vi "reLU.vi"(9 "Derivative?":bool, 11 "Input":dbl[](array[numeric])) -> (10 "Output":dbl[](array[numeric]))   [LabVIEW 2016]
panel:
  # "reLU activation function"
  # "Author: Adam Cavatassi, McGill University, 2018"
  # "False: compute reLU(x)\nTrue: compute reLU'(x)"
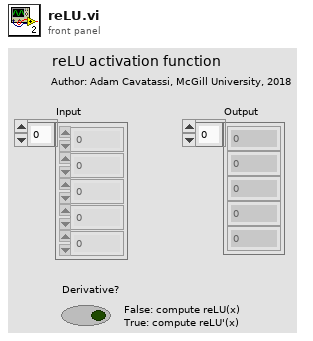
[diagram p1: front panel]
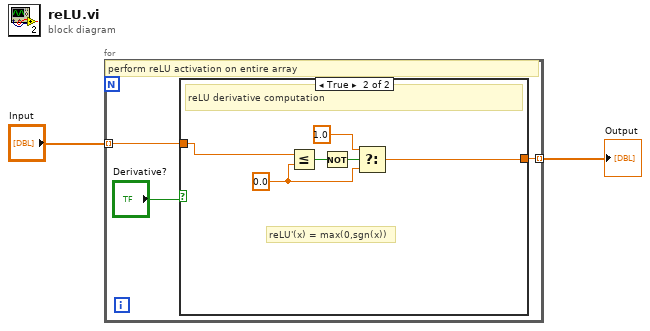
[diagram p0: block diagram]
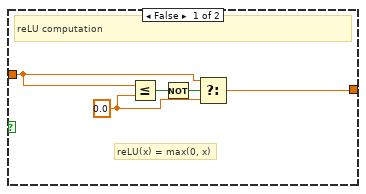
[diagram p2: hidden frame]
diagram:
  n1 = for {
    tunnel: "Input" -> [w5] mode=indexing
    tunnel: [w4] -> w1 mode=indexing
    # "perform reLU activation on entire array"
    n2 = case shown="True" "Derivative?" {
      tunnel: w5 -> [w8 w13]
      tunnel: [w6 w12] -> w4
      frame False {
        w9 = 0.0
        # "reLU(x) = max(0, x)"
        # "reLU computation"
        n3 = Less Or Equal?(x=w8, y=w9) -> (x <= y?=w10:bool)
        n4 = Not(x=w10) -> (.not. x?=w7:bool)
        n5 = Select(t=w8, s=w7, f=w9) -> (s? t:f=w6:dbl)
      }
      frame True {
        w11 = 0.0
        # "reLU'(x) = max(0,sgn(x))"
        # "reLU derivative computation"
        n6 = Less Or Equal?(x=w13, y=w11) -> (x <= y?=w16:bool)
        n7 = Not(x=w16) -> (.not. x?=w14:bool)
        n8 = Select(t=1.0, s=w14, f=w11) -> (s? t:f=w12:dbl)
      }
    }
  }
  "Output" <- w1
